vi "Write Sample Multiplier.vi"(8 "error in (no error)":errorcluster, 10 "Sample Multiplier":u32, 11 "XYGraphOverview in":refnum<class "XYGraphOverview.lvclass">) -> (0 "error out":errorcluster, 3 "XYGraphOverview out":refnum<class "XYGraphOverview.lvclass">)   [LabVIEW 2020, in "XYGraphOverview.lvlib" / "XYGraphOverview.lvclass"]
uses:
  XYGraphOverview.lvclass
  XYGraphOverview.lvclass/XYGraphOverview.ctl
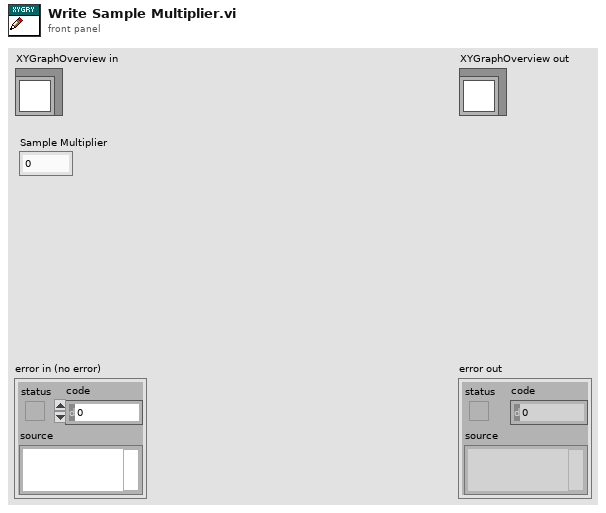
[diagram p1: front panel]
types:
  T1 = typedef "XYGraphOverview.lvlib/XYGraphOverview.lvclass/State Data.ctl" = cluster{"Sample Multiplier":u32, "Block Color":u32, "Highlight Color":u32}
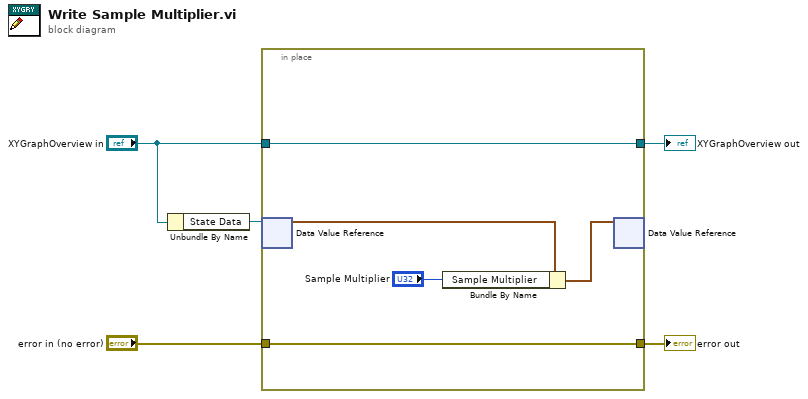
[diagram p0: block diagram]
diagram:
  n1 = Unbundle By Name("XYGraphOverview in") -> ("State Data"=w4:refnum<data-value>)
  n2 = in-place {
    in-place-border: "XYGraphOverview in" -> [w10]
    in-place-border: [w10] -> w2
    in-place-border: "error in (no error)" -> [w9]
    in-place-border: [w9] -> w1
    n3 = in-place-dvr #1(w4) -> (w8:T1)  [unwired: 1 out]
    n4 = Bundle By Name(cluster=w8, "Sample Multiplier"="Sample Multiplier") -> (w6:T1)
    n5 = in-place-dvr #1(w6) -> ()  [unwired: 2 out]
  }
  "error out" <- w1
  "XYGraphOverview out" <- w2
